vi "niFpgaDcRmsOutsideSCTL.vi"(0 "input data":fxp<+/-,32,1>, 1 "reset":bool) -> (2 "Sum result":fxp<+/-,42,11> format="%.35g", 3 "Square Sum result":fxp<+,64,10> format="%.58g", 4 "DC result":fxp<+/-,33,2> format="%.32g", 6 "RMS result":fxp<+,32,1> format="%.32g", 8 "Mean Square result":fxp<+,63,1> format="%.63g", 10 "results valid":bool)   [LabVIEW 2017]
doc: "Calculates the <B>DC (Mean)</B> and/or <B>RMS</B> values of an input signal. You also can use this VI to calculate the intermediate <B>Sum</B>, <B>Mean Square</B>, and <B>Square Sum</B> values in order to save FPGA resources."
uses:
  <vilib>/rvi/FXPMathLib/basic elements/FxpIntAccumulator/XNode/nifxpmath_IntAccumulator.xnode
  <vilib>/rvi/FXPMathLib/basic elements/FxpIntAccumulator/simVIs/DllFxpIntAccumulator_sub.vi
  <vilib>/rvi/FXPMathLib/basic elements/FxpIntAccumulator/subVIs/nifxpmath_IntAccumulator_SimConfig.ctl
  <vilib>/rvi/FXPMathLib/FxpMul/XNode/nifxpmath_Multiplier.xnode
  <vilib>/fxp/LVFixedPointOverflowPolicyTypeDef.ctl
  <vilib>/rvi/FXPMathLib/FxpSqrt/XNode/nifxpmath_Sqrt.xnode
  <vilib>/Platform/TimedLoop/XDataNode/XDataNode.xnode
  <vilib>/Platform/TimedLoop/XDataNode/nitl_modes.ctl
  <vilib>/Platform/TimedLoop/XDataNode/XDNodeRunTimeDep.lvlib
  <vilib>/Platform/TimedLoop/XDataNode/wakeup.ctl
  <vilib>/Platform/TimedLoop/XDataNode/timing_clust.ctl
  <vilib>/rvi/FXPMathLib/FxpSqrt/simVIs/DllSqrtTemp_sub.vi
  <vilib>/rvi/FXPMathLib/FxpSqrt/subVIs/nifxpmath_Sqrt_SimConfig.ctl
  <vilib>/rvi/FXPMathLib/sim/FxpSim.dll
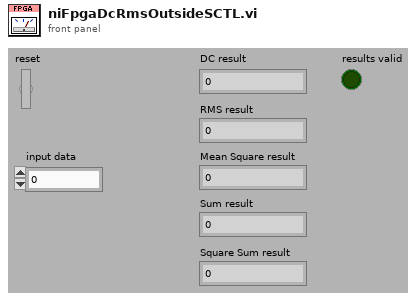
[diagram p1: front panel]
types:
  T1 = typedef "XDNodeRunTimeDep.lvlib/timing_clust.ctl" = cluster{"Expected End [f-1]":u64, "Actual End [f-1]":u64, "Finished Late? [f-1]":bool, "Expected End [i-1]":u64, "Actual End [i-1]":u64, "Finished Late? [i-1]":bool, "Expected Start [i]":u64, "Actual Start [i]":u64, "Expected Start [f]":u64, "Actual Start [f]":u64, "Source Name":string, "Structure Name":string, "Period":i64, "Deadline":i64, "Offset":i64, "Start":i64, "Priority":i32, "Timeout":i32, "Mode":T2, "Wakeup Reason":T3, "Error":errorcluster, "Source Type":string, "Secondary Source Type":string, "Global End Time":u64, "Global Start Time":u64, "Frame Duration":u64, "Iteration Duration":u64, "Assigned CPU":i32, "I/O Scan Engine Mode":u32}
  T2 = typedef "XDNodeRunTimeDep.lvlib/nitl_modes.ctl" = enum32{"No Change", "Process missed periods, maintain original phase", "Discard missed periods, maintain original phase", "Process missed periods, ignore original phase", "Discard missed periods, ignore original phase"}
  T3 = typedef "XDNodeRunTimeDep.lvlib/wakeup.ctl" = enum32{"Normal", "Aborted", "Asynchronous wakeup", "Timing source error", "Timed loop error", "Timeout"}
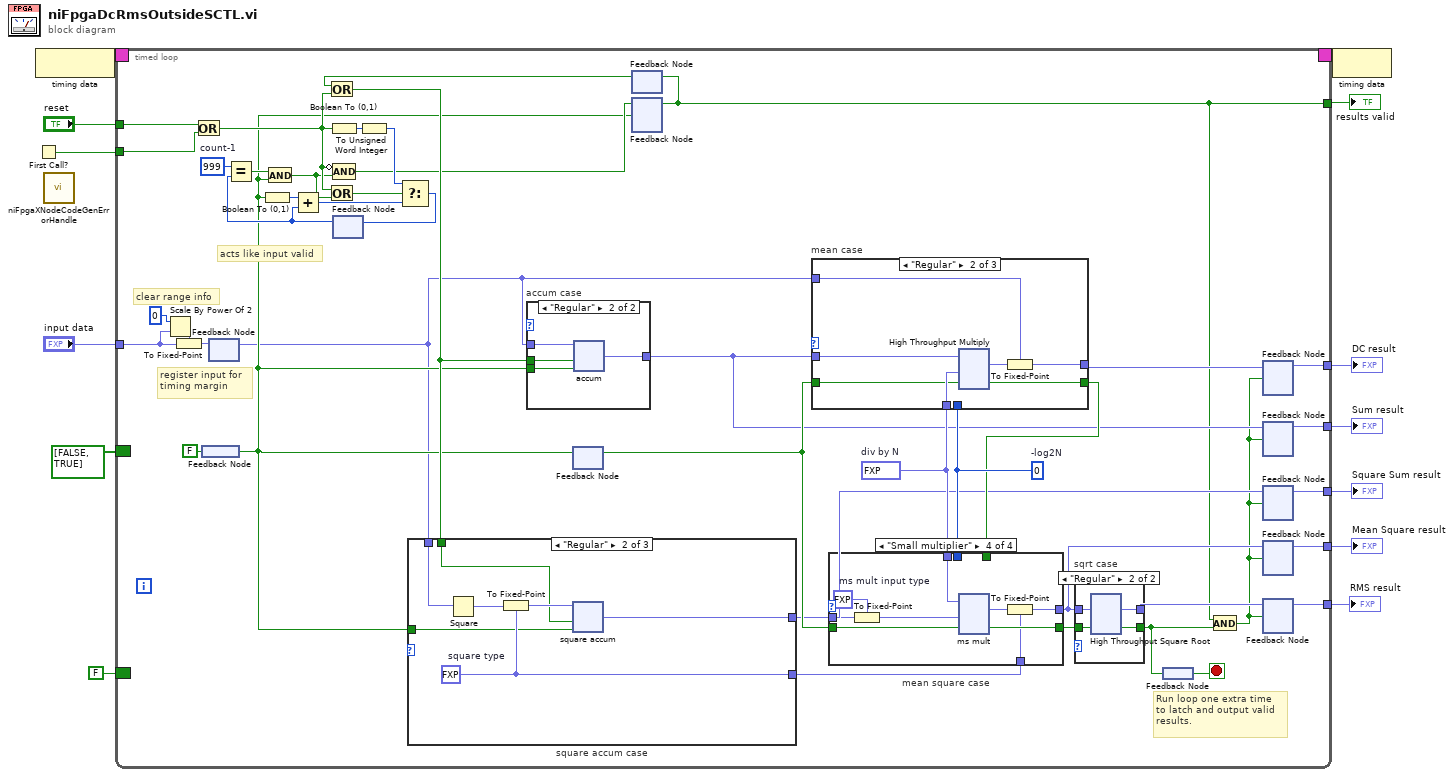
[diagram p0: block diagram]
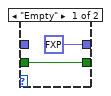
[diagram p2: hidden frame]
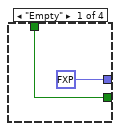
[diagram p3: hidden frame]
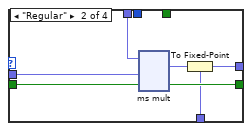
[diagram p4: hidden frame]
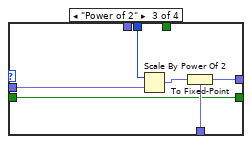
[diagram p5: hidden frame]
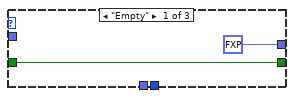
[diagram p6: hidden frame]
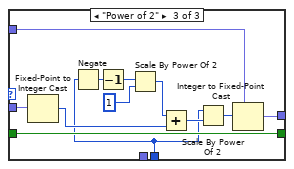
[diagram p7: hidden frame]
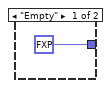
[diagram p8: hidden frame]
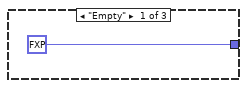
[diagram p9: hidden frame]
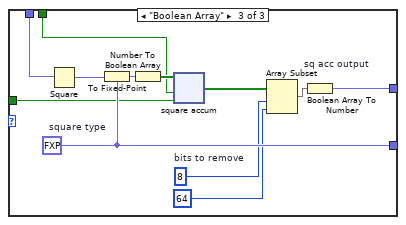
[diagram p10: hidden frame]
diagram:
  n1 = First Call?() -> (First Call?: T/F=w12:bool)
  n2 = node-c288() -> (w11:T1)
  n3 = call <vilib>:"niFpgaXNodeCodeGenErrorHandle.vi"() -> ()  [unwired: 1 in]
  n4 = timed-loop {
    tunnel: "input data" -> [w15]
    tunnel: "reset" -> [w52]
    tunnel: w12 -> [w51]
    tunnel: [w25] -> w9
    timing: w11 -> [_]
    timing-out: [_] -> w10
    border: bool[] [FALSE, TRUE] -> [_]
    tunnel: [w22] -> w7
    tunnel: [w21] -> w6
    tunnel: [w20] -> w5
    tunnel: [w19] -> w4
    tunnel: [w26] -> w3
    border: FALSE ("output valid") -> [_]
    stop <- w23 stop-if-true
    w37 = i8 0  # -log2N
    w41 = fxp<+,17,-9> 0.0010000020265579224  # div by N
    w56 = u16 999  # count-1
    # "register input for \ntiming margin"
    # "Run loop one extra time\nto latch and output valid\nresults."
    # "clear range info"
    # "acts like input valid"
    n5 = Scale By Power Of 2(n=0, x=w15) -> (x*2^n=w18:fxp<+/-,32,1>)
    n6 = To Fixed-Point(fixed-point type=w18, number=w15) -> (fixed-point=w16:fxp<+/-,32,1>)
    n7 = Or(x=w52, y=w51) -> (x .or. y?=w46:bool)
    n8 = feedback #1() -> (w33:bool)
    n9 = feedback-in #1(FALSE) -> ()
    n10 = feedback-in #2(w16) -> ()
    n11 = feedback #2() -> (w32:fxp<+/-,32,1>)  [unwired: 1 in]
    n12 = Boolean To (0,1)(Boolean=w33) -> (0, 1=w50:i16)
    n13 = Boolean To (0,1)(Boolean=w46) -> (0, 1=w55:i16)
    n14 = feedback #3() -> (w43:u16)  [unwired: 1 in]
    n15 = Equal?(x=w56, y=w43) -> (x = y?=w48:bool)
    n16 = And(x=w48, y=w33) -> (x .and. y?=w45:bool)
    n17 = Add(x=w50, y=w43) -> (x+y=w49:u16)
    n18 = Or(x=w46, y=w45) -> (x .or. y?=w47:bool)
    n19 = Compound Arithmetic op=AND(invert w46, w45) -> (w38:bool)
    n20 = To Unsigned Word Integer(number=w55) -> (unsigned 16bit integer=w54:u16)
    n21 = Select(t=w54, s=w47, f=w49) -> (s? t:f=w53:u16)
    n22 = feedback-in #3(w53) -> ()
    n23 = feedback-in #4(w33) -> ()
    n24 = feedback #4() -> (w36:bool)  [unwired: 1 in]
    n25 = feedback #5() -> (w44:bool)  [unwired: 1 in]
    n26 = Or(x=w44, y=w46) -> (x .or. y?=w40:bool)
    n27 = case "square accum case" shown="\"Regular\"" {
      selector: _ -> [_ _ _]
      tunnel: w32 -> [_ w169 w209]
      tunnel: w33 -> [_ w166 w200]
      tunnel: w40 -> [_ w165 w199]
      tunnel: [fxp<+,1,1> 0.0 ("s") w168 w201] -> w31
      tunnel: [_ w167 w208] -> w39
      frame "Empty" {
      }
      frame "Regular" {
        w167 = fxp<+,63,1> 0.0  # square type
        n28 = Square(x=w169) -> (x^2=w171:fxp<+,63,1>)
        n29 = To Fixed-Point(fixed-point type=w167, number=w171) -> (fixed-point=w170:fxp<+,63,1>)
        n30 = xnode "square accum"("x"=w170, "load (F)"=w165, "enable (T)"=w166) -> ("s"=w168:fxp<+,64,2>)  [unwired: 2 in, 1 out]
      }
      frame "Boolean Array" {
        w205 = 8  # bits to remove
        w208 = fxp<+,63,1> 0.0  # square type
        n31 = Square(x=w209) -> (x^2=w210:fxp<+,63,1>)
        n32 = To Fixed-Point(fixed-point type=w208, number=w210) -> (fixed-point=w207:fxp<+,63,1>)
        n33 = Number To Boolean Array(number=w207) -> (Boolean array=w206:bool[])
        n34 = xnode "square accum"("x"=w206, "load (F)"=w199, "enable (T)"=w200) -> ("s"=w202:bool[])  [unwired: 2 in, 1 out]
        n35 = Array Subset(array=w202, index=w205, length=64) -> (w203:bool[])
        n36 = Boolean Array To Number "sq acc output"(Boolean array=w203) -> (number=w201:fxp<+,64,10>)
      }
    }
    n37 = case "accum case" shown="\"Regular\"" {
      selector: _ -> [_ _]
      tunnel: [fxp<+/-,42,11> 0.0 ("s") w136] -> w30
      tunnel: w32 -> [_ w135]
      tunnel: w33 -> [_ w134]
      tunnel: w40 -> [_ w133]
      frame "Empty" {
      }
      frame "Regular" {
        n38 = xnode "accum"("x"=w135, "load (F)"=w133, "enable (T)"=w134) -> ("s"=w136:fxp<+/-,42,11>)  [unwired: 2 in, 1 out]
      }
    }
    n39 = feedback-in #6(w38, w33) -> ()
    n40 = feedback #6() -> (w25:bool)  [unwired: 1 in]
    n41 = feedback-in #5(w25) -> ()
    n42 = case "mean case" shown="\"Regular\"" {
      selector: _ -> [_ _ _]
      tunnel: [fxp<+/-,32,1> 0.0 ("s") w119 w122] -> w29
      tunnel: w41 -> [_ w117 _]
      tunnel: w30 -> [_ w116 w123]
      tunnel: w32 -> [_ w115 w121]
      tunnel: w36 -> [w112 w114 w131]
      tunnel: w37 -> [_ _ w120]
      tunnel: [w112 w113 w131] -> w35
      frame "Empty" {
      }
      frame "Regular" {
        n43 = xnode ("High Throughput Multiply")("x"=w116, "y"=w117, "input valid"=w114) -> ("x*y"=w118:fxp<+/-,59,2>, "output valid"=w113:bool)  [unwired: 1 in, 1 out]
        n44 = To Fixed-Point(fixed-point type=w115, number=w118) -> (fixed-point=w119:fxp<+/-,32,1>)
      }
      frame "Power of 2" {
        n45 = Fixed-Point to Integer Cast(1:w123) -> (0:w126:i64)
        n46 = Negate(x=w120) -> (-x=w130:i8)
        n47 = Decrement(x=w130) -> (x-1=w129:i8)
        n48 = Scale By Power Of 2(n=w129, x=i64 1 ("x-1")) -> (x*2^n=w127:i64)
        n49 = Add(x=w127, y=w126) -> (x+y=w124:i64)
        n50 = Scale By Power Of 2(n=w120, x=w124) -> (x*2^n=w125:i64)
        n51 = Integer to Fixed-Point Cast(fixed-point type=w121, integer=w125) -> (fixed-point=w122:fxp<+/-,32,1>)
      }
    }
    n52 = case "mean square case" shown="\"Small multiplier\"" {
      selector: _ -> [_ _ _ _]
      tunnel: [w87 w95 w96 w110] -> w42
      tunnel: w41 -> [_ w94 _ w109]
      tunnel: [fxp<+,1,1> 0.0 ("s") w92 w101 w107] -> w28
      tunnel: w39 -> [_ w91 w100 w106]
      tunnel: w31 -> [_ w90 w97 w105]
      tunnel: w37 -> [_ _ w99 _]
      tunnel: w36 -> [_ w89 w96 w102]
      tunnel: w35 -> [w87 _ _ _]
      frame "Empty" {
      }
      frame "Regular" {
        n53 = xnode ("ms mult")("x"=w94, "y"=w90, "input valid"=w89) -> ("x*y"=w93:fxp<+,64,1>, "output valid"=w95:bool)  [unwired: 1 in, 1 out]
        n54 = To Fixed-Point(fixed-point type=w91, number=w93) -> (fixed-point=w92:fxp<+,63,1>)
      }
      frame "Power of 2" {
        n55 = Scale By Power Of 2(n=w99, x=w97) -> (x*2^n=w98:fxp<+,64,10>)
        n56 = To Fixed-Point(fixed-point type=w100, number=w98) -> (fixed-point=w101:fxp<+,63,1>)
      }
      frame "Small multiplier" {
        w103 = fxp<+,34,10> 0.0  # ms mult input type
        n57 = To Fixed-Point(fixed-point type=w103, number=w105) -> (fixed-point=w104:fxp<+,34,10>)
        n58 = xnode ("ms mult")("x"=w109, "y"=w104, "input valid"=w102) -> ("x*y"=w108:fxp<+,51,1>, "output valid"=w110:bool)  [unwired: 1 in, 1 out]
        n59 = To Fixed-Point(fixed-point type=w106, number=w108) -> (fixed-point=w107:fxp<+,63,1>)
      }
    }
    n60 = case "sqrt case" shown="\"Regular\"" {
      selector: _ -> [_ _]
      tunnel: [fxp<+,1,1> 0.0 ("s") w62] -> w27
      tunnel: [w58 w61] -> w14
      tunnel: w42 -> [w58 w60]
      tunnel: w28 -> [_ w59]
      frame "Empty" {
      }
      frame "Regular" {
        n61 = xnode "High Throughput Square Root"("x"=w59, "input valid"=w60) -> ("sqrt(x)"=w62:fxp<+,32,1>, "output valid"=w61:bool)  [unwired: 1 in, 1 out]
      }
    }
    n62 = feedback-in #7(w14) -> ()
    n63 = feedback #7() -> (w23:bool)
    n64 = And(x=w25, y=w14) -> (x .and. y?=w24:bool)
    n65 = feedback #8() -> (w19:fxp<+/-,32,1>)  [unwired: 1 in]
    n66 = feedback-in #8(w29, w24) -> ()
    n67 = feedback #9() -> (w20:fxp<+/-,42,11>)  [unwired: 1 in]
    n68 = feedback-in #9(w30, w24) -> ()
    n69 = feedback #10() -> (w21:fxp<+,64,10>)  [unwired: 1 in]
    n70 = feedback-in #10(w31, w24) -> ()
    n71 = feedback #11() -> (w22:fxp<+,63,1>)  [unwired: 1 in]
    n72 = feedback-in #11(w28, w24) -> ()
    n73 = feedback #12() -> (w26:fxp<+,32,1>)  [unwired: 1 in]
    n74 = feedback-in #12(w27, w24) -> ()
  }
  "results valid" <- w9
  "DC result" <- w4
  "Mean Square result" <- w7
  "RMS result" <- w3
  "Square Sum result" <- w6
  "Sum result" <- w5
  n75 = node-c288(w10) -> ()
